vi "port_listing.vi"() -> (0 "error out":errorcluster, 2 "ports":string[](array[string]), 3 "find list":string[](array[string]))   [LabVIEW 2024]
panel:
  out "find list 2":string[](array[string])
  out "Array":errorcluster[](array[cluster])
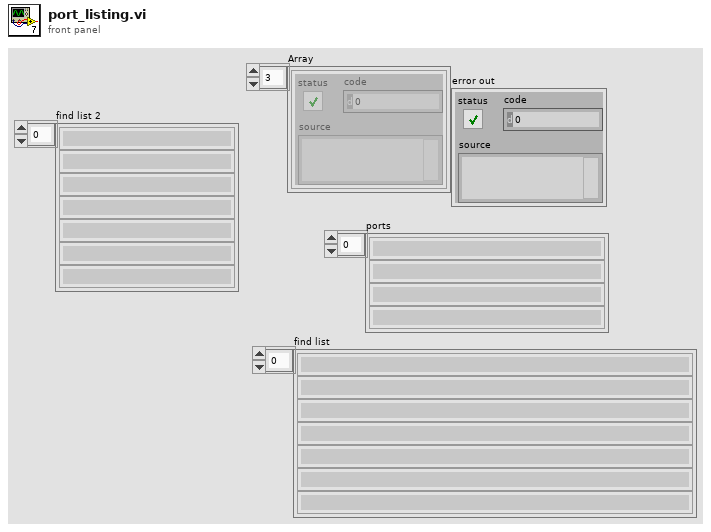
[diagram p1: front panel]
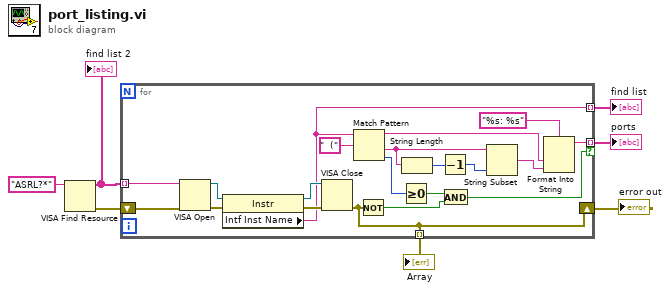
[diagram p0: block diagram]
diagram:
  n1 = VISA Find Resource(11:"ASRL?*" ("expression (\"?*\")")) -> (0:w4:errorcluster, 3:w6:string[])  [unwired: 2 in, 1 out]
  "find list 2" <- w6
  n2 = for {
    tunnel: w6 -> [w27] mode=indexing
    tunnel: [w20] -> w5 mode=indexing if=w13
    tunnel: [w12] -> w7 mode=indexing
    shift-right: [w8] -> w3
    shift-left: w4 -> [w9]
    tunnel: [w8] -> w2 mode=indexing
    n3 = VISA Open(error in (no error)=w9, VISA resource name=w27) -> (VISA resource name=w19:refnum<visa-resource-name>, error out=w17:errorcluster)  [unwired: 3 in]
    n4 = property class="Instr"(reference=w19, error in=w17) -> (reference out=w26:refnum<visa-resource-name>, error out=w18:errorcluster, "Intf Inst Name"=w12:string)
    n5 = VISA Close(VISA resource name=w26, error in (no error)=w18) -> (error out=w8:errorcluster)
    n6 = Match Pattern(string=w12, regular expression="  (") -> (before substring=w10:string, after substring=w23:string, offset past match=w16:i32)  [unwired: 1 in, 1 out]
    n7 = Not(x=w8) -> (.not. x?=w15:bool)
    n8 = Greater Or Equal To 0?(x=w16) -> (x >= 0?=w14:bool)
    n9 = String Length(string=w23) -> (length=w22:i32)
    n10 = Decrement(x=w22) -> (x-1=w21:i32)
    n11 = And(x=w14, y=w15) -> (x .and. y?=w13:bool)
    n12 = String Subset(string=w23, length (rest)=w21) -> (substring=w11:string)  [unwired: 1 in]
    n13 = Format Into String(format string="%s: %s", w10, w11) -> (resulting string=w20:string)  [unwired: 2 in, 1 out]
  }
  "error out" <- w3
  "ports" <- w5
  "find list" <- w7
  "Array" <- w2
